vi "数码管显示.vi"() -> ()   [LabVIEW 2013]
panel:
  in  "停止":bool
  in  "数字显示":u16(ring) items=["0", "1", "2", "3", "4", "5", "6", "7", "8", "9"]
  out "数码管显示":T1
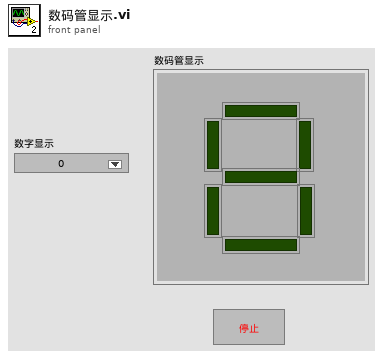
[diagram p1: front panel]
types:
  T1 = cluster{"布尔":bool, "布尔 2":bool, "布尔 3":bool, "布尔 4":bool, "布尔 3":bool, "布尔 5":bool, "布尔 6":bool}
  T2 = cluster{"[0]":bool, "[1]":bool, "[2]":bool, "[3]":bool, "[4]":bool, "[5]":bool, "[6]":bool}
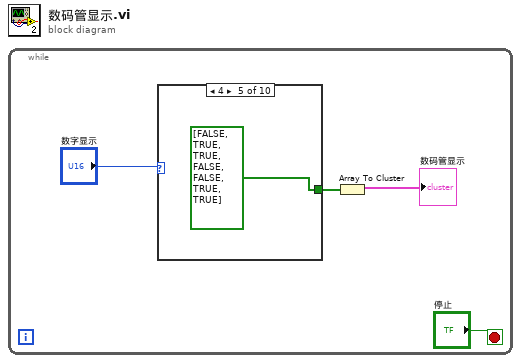
[diagram p0: block diagram]
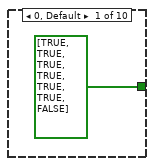
[diagram p2: hidden frame]
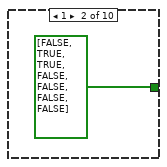
[diagram p3: hidden frame]
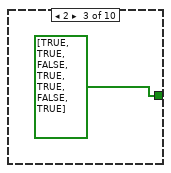
[diagram p4: hidden frame]
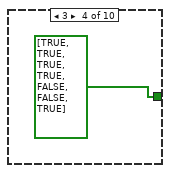
[diagram p5: hidden frame]
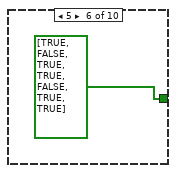
[diagram p6: hidden frame]
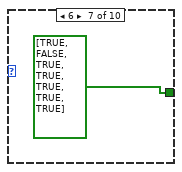
[diagram p7: hidden frame]
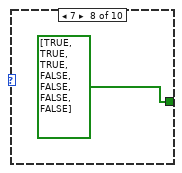
[diagram p8: hidden frame]
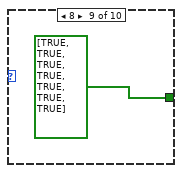
[diagram p9: hidden frame]
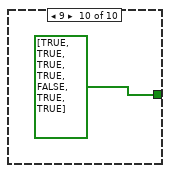
[diagram p10: hidden frame]
diagram:
  n1 = while {
    stop <- "停止" stop-if-true
    n2 = case shown="4" "数字显示" {
      tunnel: [bool[] [TRUE, TRUE, TRUE, TRUE, TRUE, TRUE, FALSE] bool[] [FALSE, TRUE, TRUE, FALSE, FALSE, FALSE, FALSE] bool[] [TRUE, TRUE, FALSE, TRUE, TRUE, FALSE, TRUE] bool[] [TRUE, TRUE, TRUE, TRUE, FALSE, FALSE, TRUE] bool[] [FALSE, TRUE, TRUE, FALSE, FALSE, TRUE, TRUE] bool[] [TRUE, FALSE, TRUE, TRUE, FALSE, TRUE, TRUE] bool[] [TRUE, FALSE, TRUE, TRUE, TRUE, TRUE, TRUE] bool[] [TRUE, TRUE, TRUE, FALSE, FALSE, FALSE, FALSE] bool[] [TRUE, TRUE, TRUE, TRUE, TRUE, TRUE, TRUE] bool[] [TRUE, TRUE, TRUE, TRUE, FALSE, TRUE, TRUE]] -> w2
      frame 0, Default {
      }
      frame 1 {
      }
      frame 2 {
      }
      frame 3 {
      }
      frame 4 {
      }
      frame 5 {
      }
      frame 6 {
      }
      frame 7 {
      }
      frame 8 {
      }
      frame 9 {
      }
    }
    n3 = Array To Cluster(array=w2) -> (cluster=→"数码管显示":T2)
  }
